vi "runtime io test.vi"() -> (0 "no error":errorcluster)   [LabVIEW 2013, in "tdms logger tests.lvlib"]
uses:
  tdms logger tests.lvlib
  execution/TDMS datalogger runtime.lvclass
  <vilib>/NI/Tag Bus/tag/tag descriptor.lvclass/tag descriptor.ctl
  <vilib>/NI/Tag Bus/table/data polymorphs/write one/write Double.vi
  <vilib>/NI/Tag Bus/tag/read tag name.vi
  <vilib>/NI/Tag Bus/tag/read data type.vi
  <vilib>/NI/Tag Bus/dictionary/data dictionary.lvclass
  <vilib>/NI/Tag Bus Module Framework/channel/TBM channel.lvclass
  <vilib>/NI/Tag Bus/table/data table.lvlib
panel:
  # "This is expected to remain false until you write code for input"
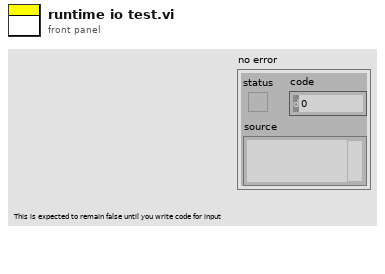
[diagram p1: front panel]
types:
  T1 = typedef "TBM channel.lvclass/data tables.ctl" = cluster{"input data":T2, "processing parameter":T2, "processing result":T2, "output data":T2}
  T2 = typedef "tag bus.lvlib/dictionary table pair.ctl" = cluster{"data dictionary":refnum<class "data dictionary.lvclass">, "data table":T3}
  T3 = typedef "tag bus.lvlib/data table.lvlib/data table.ctl" = cluster{"Double":dbl[], "Single":sgl[], "I64":i64[], "I32":i32[], "I16":i16[], "I8":i8[], "U64":u64[], "U32":u32[], "U16":u16[], "U8":u8[], "Boolean":bool[], "String":string[], "Array of Double":cluster{"DBL Array":dbl[]}[], "Array of Single":cluster{"SGL Array":sgl[]}[], "Array of I64":cluster{"I64 Array":i64[]}[], "Array of I32":cluster{"I32 Array":i32[]}[], "Array of I16":cluster{"I16 Array":i16[]}[], "Array of I8":cluster{"I8 Array":i8[]}[], "Array of U64":cluster{"U64 Array":u64[]}[], "Array of U32":cluster{"U32 Array":u32[]}[], "Array of U16":cluster{"U16 Array":u16[]}[], "Array of U8":cluster{"U8 Array":u8[]}[], "Array of Boolean":cluster{"Boolean Array":bool[]}[], "Array of String":cluster{"String Array":string[]}[]}
  T4 = typedef "tag bus.lvlib/tag descriptor.lvclass/Data Type.ctl" = enum16{"Double", "Single", "I64", "I32", "I16", "I8", "U64", "U32", "U16", "U8", "Boolean", "String", "Array of Double", "Array of Single", "Array of I64", "Array of I32", "Array of I16", "Array of I8", "Array of U64", "Array of U32", "Array of U16", "Array of U8", "Array of Boolean", "Array of String"}
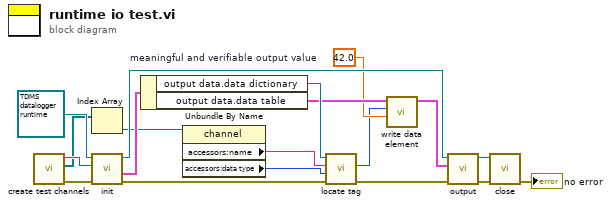
[diagram p0: block diagram]
diagram:
  w8 = 42.0  # meaningful and verifiable output value
  n1 = call "create test channels.vi"() -> ("error out"=w1:errorcluster, "chans"=w2:refnum<class "TBM channel.lvclass">[], "TDMS datalogger configuration out"=w3:refnum<class "TDMS datalogger configuration.lvclass">)  [unwired: 8 in, 1 out]
  n2 = Index Array(array=w2) -> (element=w4:refnum<class "TBM channel.lvclass">)  [unwired: 1 in]
  n3 = call-dynamic "init.vi"("error in"=w1, "TBM module configuration in"=w3, "TDMS datalogger runtime in"=refnum<class "TDMS datalogger runtime.lvclass"> refnum ("TDMS datalogger runtime")) -> ("error out"=w11:errorcluster, "data allocations"=w15:T1, "TDMS datalogger runtime out"=w16:refnum<class "TDMS datalogger runtime.lvclass">)  [unwired: 5 in, 1 out]
  n4 = Unbundle By Name(w15) -> ("output data.data dictionary"=w14:refnum<class "data dictionary.lvclass">, "output data.data table"=w10:T3)
  n5 = property class="channel"(reference=w4) -> ("accessors:name"=w13:string, "accessors:data type"=w12:T4)  [unwired: 1 in, 2 out]
  n6 = call <vilib>:"locate tag.vi"("error in"=w11, "data type"=w12, "name"=w13, "data dictionary in"=w14) -> ("error out"=w6:errorcluster, "index"=w5:i32)  [unwired: 5 in, 1 out]
  n7 = call-poly <vilib>:"write data element.vi"("value"=w8, "index"=w5, "data table in"=w10) -> ("data table out"=w9:T3)  [unwired: 8 in]
  n8 = call-dynamic "output.vi"("error in"=w6, "data table in"=w9, "TDMS datalogger runtime in"=w16) -> ("error out"=w17:errorcluster, "TDMS datalogger runtime out"=w18:refnum<class "TDMS datalogger runtime.lvclass">)  [unwired: 6 in, 1 out]
  n9 = call-dynamic "close.vi"("error in"=w17, "TDMS datalogger runtime in"=w18) -> ("error out"=→"no error":errorcluster)  [unwired: 9 in]
